vi "Open_New_WorkSheet.vi"(0 "Excel._Workbook":refnum<k7>, 1 "Page index":i32=1, 5 "SheetName":string, 11 "error in (no error)":errorcluster) -> (4 "Excel._Worksheet":refnum<k7>, 15 "error out":errorcluster)   [LabVIEW 2014]
doc: "Opens a new WorkSheet. Takes a Workbook Refnum as input."
panel:
  in  "Excel._Worksheet":refnum<k7>
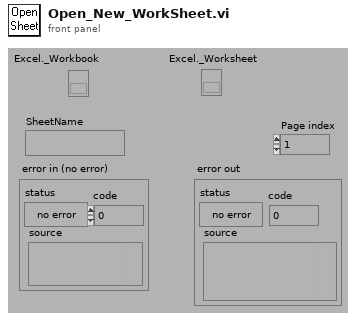
[diagram p1: front panel]
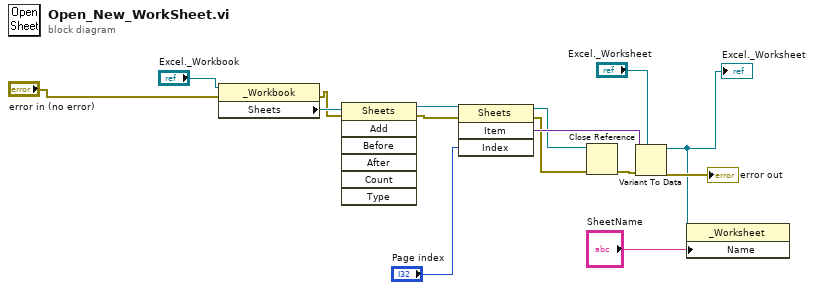
[diagram p0: block diagram]
diagram:
  n1 = property class="_Workbook"(reference="Excel._Workbook", error in="error in (no error)") -> (error out=w1:errorcluster, "Sheets"=w4:refnum<k7>)  [unwired: 1 out]
  n2 = invoke class="Sheets" method="Add"(reference=w4, error in=w1) -> (reference out=w3:refnum<k7>, error out=w2:errorcluster)  [unwired: 5 in, 5 out]
  n3 = invoke class="Sheets" method="Item"(reference=w3, error in=w2, "Index"="Page index") -> (reference out=w8:refnum<k7>, error out=w14:errorcluster, "Item"=w15:variant)  [unwired: 1 in, 1 out]
  n4 = Close Reference(reference=w8, error in (no error)=w14) -> (error out=w13:errorcluster)
  n5 = Variant To Data(error in=w13, type="Excel._Worksheet", Variant=w15) -> (data=w7:refnum<k7>, error out=→"error out":errorcluster)
  "Excel._Worksheet" <- w7
  n6 = property class="_Worksheet"(reference=w7, "Name"="SheetName") -> ()  [unwired: 1 in, 2 out]
